vi "Write Instrument Info.vi"(8 "error in (no error)":errorcluster, 10 "Instrument Info":string, 11 "Cal Standard Base in":refnum<class "Cal Standard Base.lvclass">) -> (0 "error out":errorcluster, 3 "Cal Standard Base out":refnum<class "Cal Standard Base.lvclass">)   [LabVIEW 2023, in "RFFixtureCharact.Instruments.lvlib" / "Cal Standard Base.lvclass"]
uses:
  Cal Standard Base.lvclass
  Cal Standard Base.lvclass/Cal Standard Base.ctl
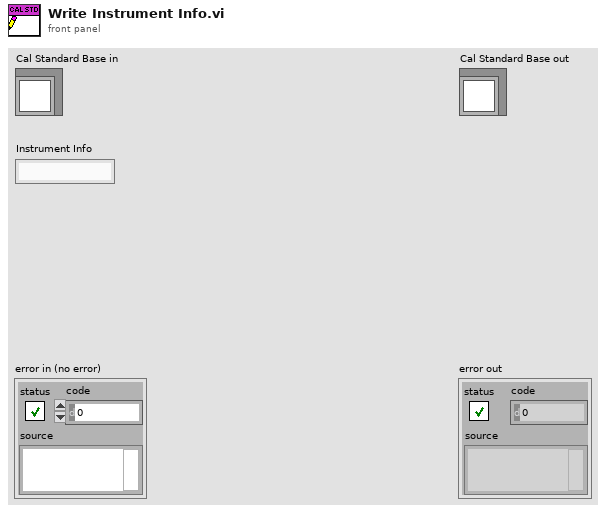
[diagram p1: front panel]
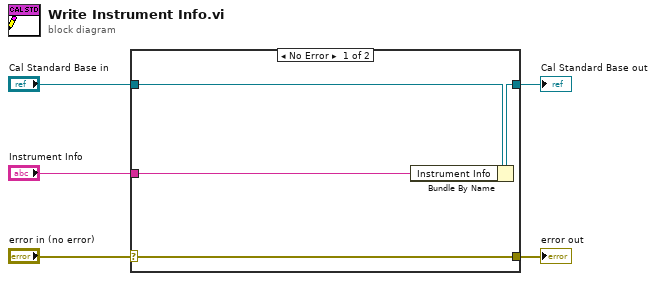
[diagram p0: block diagram]
diagram:
  n1 = case shown="No Error" "error in (no error)" {
    selector: "error in (no error)" -> [w9 w10]
    tunnel: [w9 w10] -> w4
    tunnel: [w7 w11] -> w2
    tunnel: "Cal Standard Base in" -> [w8 w11]
    tunnel: "Instrument Info" -> [w6 _]
    frame No Error {
      n2 = Bundle By Name(cluster=w8, "Instrument Info"=w6) -> (w7:refnum<class "Cal Standard Base.lvclass">)
    }
    frame Error {
    }
  }
  "error out" <- w4
  "Cal Standard Base out" <- w2
